vi "Get Tuner Gains.vi"(8 "error in (no error)":errorcluster, 11 "RTL-SDR in":refnum<class "RTL-SDR.lvclass">) -> (0 "error out":errorcluster, 1 "function return":i32, 2 "Supported Gains":dbl[](array[numeric]), 3 "RTL-SDR out":refnum<class "RTL-SDR.lvclass">)   [LabVIEW 2015, in "RTL-SDR.lvclass"]
uses:
  RTL-SDR.lvclass
panel:
  in  "Gains Buffer":i32[](array[numeric])
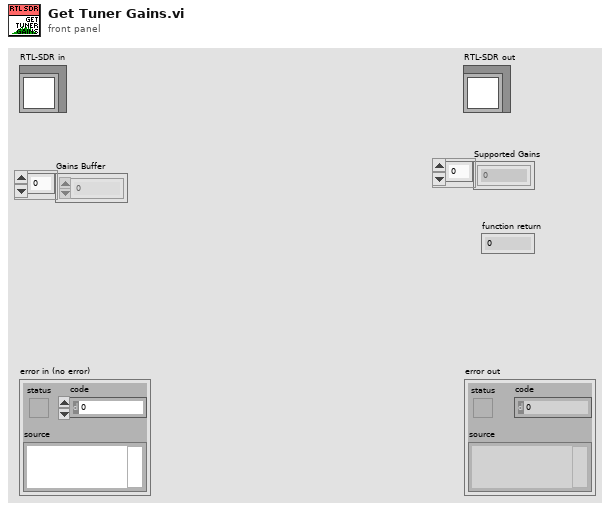
[diagram p1: front panel]
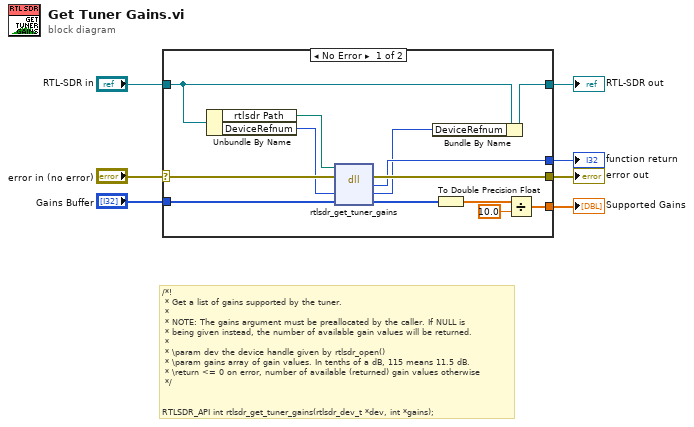
[diagram p0: block diagram]
diagram:
  # "/*!\n * Get a list of gains supported by the tuner.\n *\n * NOTE: The gains argument must be preallocated by the caller. If NULL is\n * being given instead, the number of available gain values will be returned.\n *\n * \\param dev the device handle given by rtlsdr_open()\n * \\param gains array of gain values. In tenths of a dB, 115 means 11.5 dB.\n * \\return <= 0 on error, number of available (returned) gain values otherwise\n */\n\n\nRTLSDR_API int rtlsdr_get_tuner_gains(rtlsdr_dev_t *dev, int *gains);"
  n1 = case shown="No Error" "error in (no error)" {
    selector: "error in (no error)" -> [w20 w22]
    tunnel: [w19 w22] -> w6
    tunnel: [w14 w21] -> w4
    tunnel: "RTL-SDR in" -> [w17 w21]
    tunnel: [w18 _] -> w3
    tunnel: "Gains Buffer" -> [w12 _]
    tunnel: [w8 _] -> w1
    frame No Error {
      n2 = Unbundle By Name(w17) -> ("rtlsdr Path"=w16:path, "DeviceRefnum"=w15:u64)
      n3 = dll-call lib="C:/Users/Ivan/Desktop/D-23-09-24 (RTL-SDR)/Project (Pelleng-SDR)/RTL-SDR Class/dll/rtlsdr.*" fn="rtlsdr_get_tuner_gains"(path in=w16, error in=w20, "DeviceRefnum"=w15, "Gains"=w12) -> (error out=w19:errorcluster, "return type"=w18:i32, "DeviceRefnum"=w13:u64, "Gains"=w9:i32[])  [unwired: 1 in, 1 out]
      n4 = Bundle By Name(cluster=w17, "DeviceRefnum"=w13) -> (w14:refnum<class "RTL-SDR.lvclass">)
      n5 = To Double Precision Float(number=w9) -> (double precision float=w10:dbl[])
      n6 = Divide(x=w10, y=10.0) -> (x/y=w8:dbl[])
    }
    frame Error {
    }
  }
  "error out" <- w6
  "RTL-SDR out" <- w4
  "Supported Gains" <- w1
  "function return" <- w3
